vi "IR121129 Traitement Enr Spectre_SD.vi"(1 "resultat_input":dbl[](array[numeric])=array[24576 elements]) -> (0 "Sig et ref -BG et BGsig et ref":dbl[][](array[numeric]))   [LabVIEW 2015]
uses:
  globalVarSD.vi
panel:
  out "Graphe":dbl[](graph)
  out "BGref":dbl[](array[numeric])
  out "BGSig":dbl[](array[numeric])
  out "Ref-BG":dbl[](array[numeric])
  out "Sig-BG":dbl[](array[numeric])
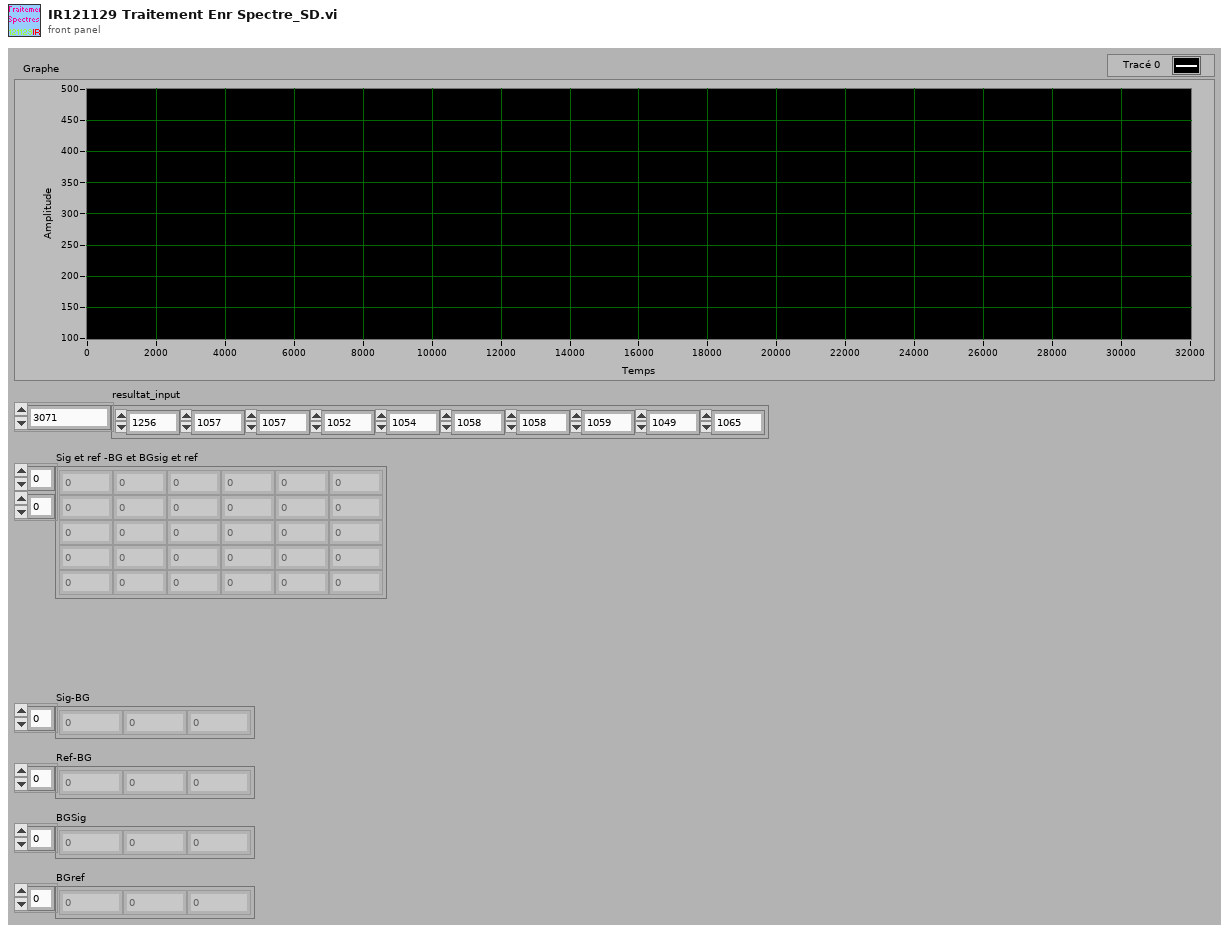
[diagram p1: front panel]
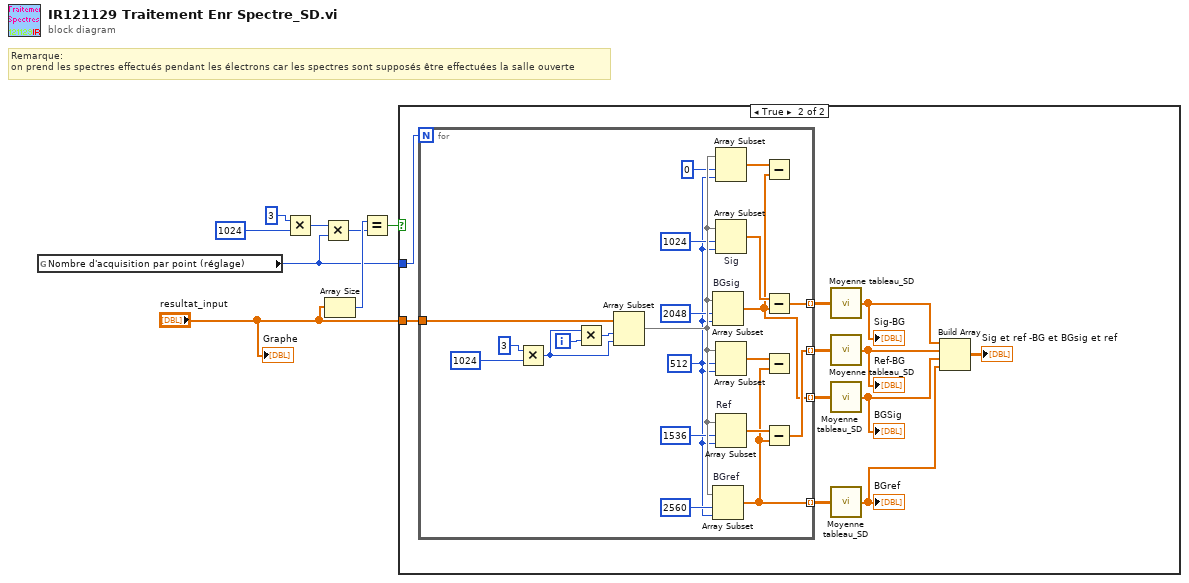
[diagram p0: block diagram]
diagram:
  # "Remarque: \non prend les spectres effectués pendant les électrons car les spectres sont supposés être effectuées la salle ouverte"
  n1 = global read "globalVarSD.vi" "Nombre d'acquisition par point (réglage)"() -> (w1:u32)
  n2 = Multiply(x=3, y=1024) -> (x*y=w6:i32)
  n3 = Multiply(x=w6, y=w1) -> (x*y=w4:u32)
  n4 = Array Size(array="resultat_input") -> (size(s)=w5:i32)
  n5 = Equal?(x=w5, y=w4) -> (x = y?=w3:bool)
  n6 = case shown="True" w3 {
    tunnel: "resultat_input" -> [_ w19]
    tunnel: w1 -> [_ w18]
    frame False {
    }
    frame True {
      n7 = for {
        N: w18 -> [_]
        tunnel: w19 -> [w38]
        tunnel: [w24] -> w17 mode=indexing
        tunnel: [w23] -> w16 mode=indexing
        tunnel: [w22] -> w15 mode=indexing
        tunnel: [w21] -> w14 mode=indexing
        i -> [w28]
        w20 = 512 ("indice")
        n8 = Multiply(x=3, y=1024) -> (x*y=w36:i32)
        n9 = Multiply(x=w36, y=w28) -> (x*y=w37:i32)
        n10 = Array Subset(array=w38, index=w37, length=w36) -> (w31:dbl[])
        n11 = Array Subset "BGsig"(array=w31, index=2048 ("indice"), length=w20) -> (w22:dbl[])
        n12 = Array Subset "BGref"(array=w31, index=2560 ("indice"), length=w20) -> (w21:dbl[])
        n13 = Array Subset(array=w31, index=0 ("indice"), length=w20) -> (w33:dbl[])
        n14 = Array Subset "Sig"(array=w31, index=1024 ("indice"), length=w20) -> (w35:dbl[])
        n15 = Array Subset(array=w31, index=w20, length=w20) -> (w32:dbl[])
        n16 = Array Subset "Ref"(array=w31, index=1536 ("indice"), length=w20) -> (w34:dbl[])
        n17 = Subtract(x=w33, y=w22) -> ()  [unwired: 1 out]
        n18 = Subtract(x=w35, y=w22) -> (x-y=w24:dbl[])
        n19 = Subtract(x=w32, y=w21) -> ()  [unwired: 1 out]
        n20 = Subtract(x=w34, y=w21) -> (x-y=w23:dbl[])
      }
      n21 = call "Moyenne tableau_SD.vi"("Signaux"=w17) -> ("Tableau"=w13:dbl[])
      "Sig-BG" <- w13
      n22 = call "Moyenne tableau_SD.vi"("Signaux"=w16) -> ("Tableau"=w12:dbl[])
      "Ref-BG" <- w12
      n23 = call "Moyenne tableau_SD.vi"("Signaux"=w15) -> ("Tableau"=w11:dbl[])
      "BGSig" <- w11
      n24 = call "Moyenne tableau_SD.vi"("Signaux"=w14) -> ("Tableau"=w10:dbl[])
      "BGref" <- w10
      n25 = Build Array(w13, w12, w11, w10) -> (→"Sig et ref -BG et BGsig et ref":dbl[][])
    }
  }
  "Graphe" <- "resultat_input"
